vi "autonomia - dojazd do punktow.vi"() -> ()   [LabVIEW 2012]
uses:
  <vilib>/robotics/Starter Kit/1.0/9631 Host Interface/NI_Robotics_Starter Kit Host_9631_1.0.lvclass
  <vilib>/robotics/Starter Kit/Host Interface/NI_Robotics_Starter Kit Host.lvclass
panel:
  in  "stop":bool
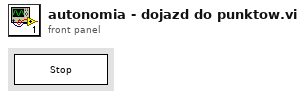
[diagram p1: front panel]
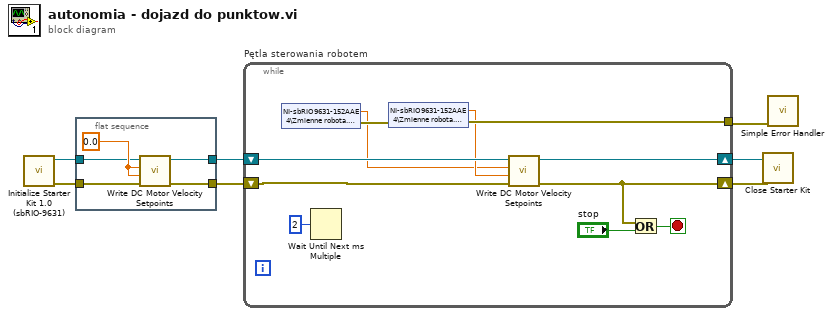
[diagram p0: block diagram]
diagram:
  n1 = call <vilib>:"Initialize Starter Kit 1.0 (sbRIO-9631).vi"() -> ("error out"=w5:errorcluster, "FPGA starter kit host 1.0 out"=w4:refnum<class "NI_Robotics_Starter Kit Host_9631_1.0.lvclass">)  [unwired: 10 in]
  n2 = flat-sequence {
    tunnel: w4 -> [w11]
    tunnel: w5 -> [w8]
    tunnel: [w10] -> w7
    tunnel: [w9] -> w6
    frame #0 {
      w12 = 0.0 ("left ccw motor velocity (rad/s)")
      n3 = call <vilib>:"Write DC Motor Velocity Setpoints.vi"("error in (no error)"=w8, "right motor ccw velocity (rad/s)"=w12, "left motor ccw velocity (rad/s)"=w12, "starter kit host in"=w11) -> ("error out"=w9:errorcluster, "starter kit host out"=w10:refnum<class "NI_Robotics_Starter Kit Host_9631_1.0.lvclass">)  [unwired: 6 in]
    }
  }
  n4 = while "Pętla sterowania robotem" {
    shift-right: [w15] -> w2
    shift-left: w6 -> [w19]
    shift-right: [w16] -> w3
    shift-left: w7 -> [w20]
    tunnel: [w18] -> w1
    stop <- w23 stop-if-true
    n5 = shared-variable "NI-sbRIO9631-152AAE4\\Zmienne robota.lvlib\\Vl[rps]"() -> (w13:dbl, error out=w14:errorcluster)  [unwired: 1 in]
    n6 = Wait Until Next ms Multiple(millisecond multiple=u32 2) -> ()  [unwired: 1 out]
    n7 = shared-variable "NI-sbRIO9631-152AAE4\\Zmienne robota.lvlib\\Vr[rps]"(error in=w14) -> (w17:dbl, error out=w18:errorcluster)
    n8 = call <vilib>:"Write DC Motor Velocity Setpoints.vi"("error in (no error)"=w19, "right motor ccw velocity (rad/s)"=w17, "left motor ccw velocity (rad/s)"=w13, "starter kit host in"=w20) -> ("error out"=w15:errorcluster, "starter kit host out"=w16:refnum<class "NI_Robotics_Starter Kit Host_9631_1.0.lvclass">)  [unwired: 6 in]
    n9 = Or(x=w15, y="stop") -> (x .or. y?=w23:bool)
  }
  n10 = call-dynamic "Close Starter Kit.vi"("error in (no error)"=w2, "starter kit host in"=w3) -> ()  [unwired: 9 in, 1 out]
  n11 = call <vilib>:"Simple Error Handler.vi"("error in (no error)"=w1) -> ()  [unwired: 4 in, 5 out]
